vi "SetupSpectrumAnalyzerForCal.vi"(0 "VISA Refnum in":refnum<visa-resource-name>="TCPIP0::169.254.70.120::inst0::INSTR", 1 "Select INST":string(combo)="INST SA", 2 "IsPSA(t)":bool=TRUE, 3 "RBW":string="3", 5 "RefLvl":string="0", 6 "ATT":dbl format="%#_13g", 9 "AVG Count":i32=16, 10 "Internal Preamp (0: Off)":i32(ring)=2 items=["Off", "Low Band", "Full Range"], 11 "error in (no error)":errorcluster, 12 "SET CF (MHz)":dbl=20000.0, 14 "Span(MHz)":dbl=0.1 format="%#_13g") -> (4 "Session Out":refnum<visa-resource-name>="TCPIP0::169.254.70.120::inst0::INSTR", 15 "error out":errorcluster {"code" format="%.0x"})   [LabVIEW 2018]
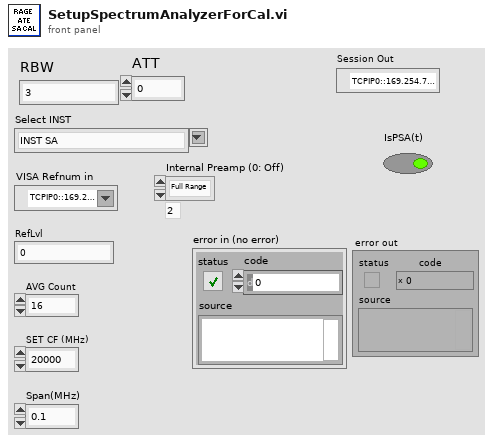
[diagram p1: front panel]
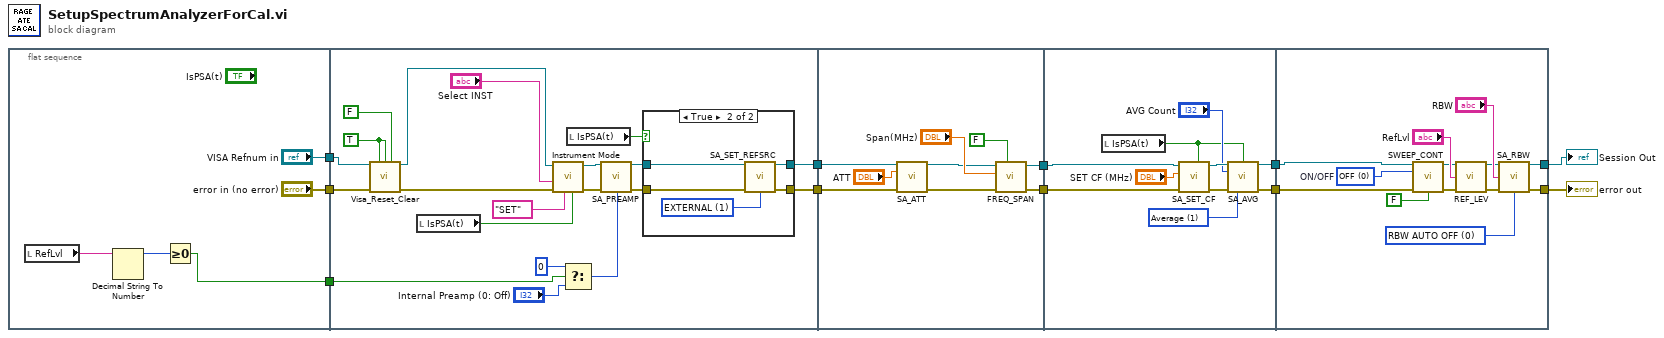
[diagram p0: block diagram]
diagram:
  n1 = flat-sequence {
    tunnel: ["VISA Refnum in"] -> w11
    tunnel: ["error in (no error)"] -> w10
    tunnel: [w12] -> w1
    tunnel: w10 -> [w33]
    tunnel: w11 -> [w34]
    tunnel: [w25] -> w9
    tunnel: [w21] -> w8
    tunnel: w1 -> [w17]
    tunnel: w9 -> [w51]
    tunnel: w8 -> [w50]
    tunnel: [w45] -> w7
    tunnel: [w44] -> w6
    tunnel: w7 -> [w58]
    tunnel: w6 -> [w57]
    tunnel: [w55] -> w5
    tunnel: [w54] -> w4
    tunnel: w5 -> [w75]
    tunnel: w4 -> [w73]
    tunnel: [w64] -> w3
    tunnel: [w63] -> w2
    frame #0 {
      n2 = local read "RefLvl"() -> (w14:string)
      n3 = Decimal String To Number(string=w14) -> (number=w13:i32)  [unwired: 2 in, 1 out]
      n4 = Greater Or Equal To 0?(x=w13) -> (x >= 0?=w12:bool)
    }
    frame #1 {
      w31 = TRUE ("Send *CLS")
      n5 = call "Visa_Reset_Clear.vi"("VISA resource name"=w34, "Send *CLS"=w31, "Restore Defaults"=w31, "Close VISA session"=FALSE, "error in (no error)"=w33) -> ("VISA resource name Out"=w27:refnum<visa-resource-name>, "error out"=w28:errorcluster)  [unwired: 9 in]
      n6 = local read "IsPSA(t)"() -> (w26:bool)
      n7 = call "Instrument Mode.vi"("SKIP(T)"=w26, "SET/GET"="SET", "error in"=w28, "Select INST"="Select INST", "Session In"=w27) -> ("error out"=w35:errorcluster, "Session Out"=w36:refnum<visa-resource-name>)  [unwired: 4 in, 1 out]
      n8 = Select(t=0, s=w17, f="Internal Preamp (0: Off)") -> (s? t:f=w19:i32)
      n9 = local read "IsPSA(t)"() -> (w23:bool)
      n10 = call "SA_PREAMP.vi"("VISA resource name"=w36, "error in (no error)"=w35, "Internal Preamp (0: Off)"=w19) -> ("VISA resource name out"=w24:refnum<visa-resource-name>, "error out"=w22:errorcluster)  [unwired: 11 in]
      n11 = case shown="True" w23 {
        tunnel: [w38 w43] -> w25
        tunnel: w24 -> [w38 w42]
        tunnel: w22 -> [w37 w41]
        tunnel: [w37 w40] -> w21
        frame False {
        }
        frame True {
          w39 = 1 items=["INTERNAL", "EXTERNAL", "SENSE(XA Series)", "PULS(XA Series)"] ("REF_SRC [INT|EXT]")
          n12 = call "SA_SET_REFSRC.vi"("Session In"=w42, "error in"=w41, "REF_SRC [INT|EXT]"=w39) -> ("Session Out"=w43:refnum<visa-resource-name>, "error out"=w40:errorcluster)  [unwired: 10 in, 1 out]
        }
      }
    }
    frame #2 {
      n13 = call "SA_ATT.vi"("Session In"=w51, "ATT"="ATT", "error in"=w50) -> ("Session Out"=w46:refnum<visa-resource-name>, "error out"=w48:errorcluster)  [unwired: 9 in, 2 out]
      n14 = call "FREQ_SPAN.vi"("RO (T)"=FALSE, "error in"=w48, "Span(MHz)"="Span(MHz)", "Session In"=w46) -> ("error out"=w45:errorcluster, "Session Out"=w44:refnum<visa-resource-name>)  [unwired: 5 in, 1 out]
    }
    frame #3 {
      w56 = 1 items=["Clear Write", "Average", "Maximum Hold", "Minimum Hold"] ("Trace Type (0: Clear Write)")
      n15 = local read "IsPSA(t)"() -> (w53:bool)
      n16 = call "SA_SET_CF.vi"("IsPSA(t)"=w53, "error in"=w58, "SET CF ()"="SET CF (MHz)", "Session In"=w57) -> ("error out"=w62:errorcluster, "Session Out"=w61:refnum<visa-resource-name>)  [unwired: 5 in, 1 out]
      n17 = call "SA_AVG.vi"("Session In"=w61, "IsPSA(t)"=w53, "AVG Count"="AVG Count", "error in"=w62, "Trace Type (0: Clear Write)"=w56) -> ("Session Out"=w55:refnum<visa-resource-name>, "error out"=w54:errorcluster)  [unwired: 9 in]
    }
    frame #4 {
      w65 = 0 items=["RBW AUTO OFF", "RBW AUTO ON"] ("RBW AUTO")
      w74 = u16 0 items=["OFF", "ON"]  # ON/OFF
      n18 = call "SWEEP_CONT.vi"("Session In"=w75, "ON/OFF"=w74, "error in"=w73, "RO (T)"=FALSE) -> ("Session Out"=w70:refnum<visa-resource-name>, "error out"=w69:errorcluster)  [unwired: 9 in, 1 out]
      n19 = call "REF_LEV.vi"("Session In"=w70, "RefLvl"="RefLvl", "error in"=w69) -> ("Session Out"=w67:refnum<visa-resource-name>, "error out"=w66:errorcluster)  [unwired: 9 in, 2 out]
      n20 = call "SA_RBW.vi"("Session In"=w67, "RBW(Hz)"="RBW", "error in"=w66, "RBW AUTO"=w65) -> ("Session Out"=w64:refnum<visa-resource-name>, "error out"=w63:errorcluster)  [unwired: 7 in, 3 out]
    }
  }
  "Session Out" <- w3
  "error out" <- w2
